vi "Generate Data_2.vi"(11 "Input":i32) -> (3 "Array out":dbl[][](array[numeric]))   [LabVIEW 2010]
panel:
  out "Waveform Graph":dbl[](graph)
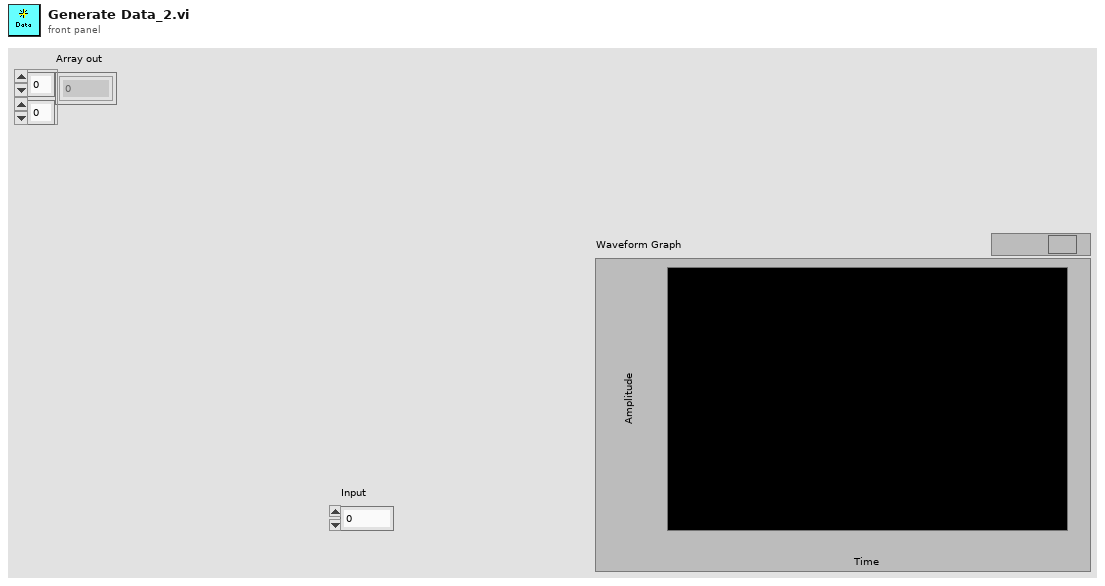
[diagram p1: front panel]
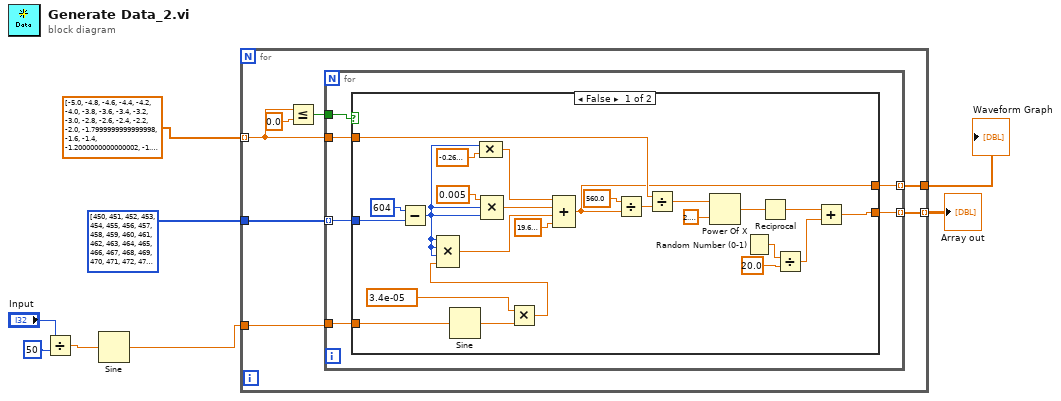
[diagram p0: block diagram]
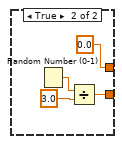
[diagram p2: hidden frame]
diagram:
  n1 = Divide(x="Input", y=50) -> (x/y=w2:dbl)
  n2 = Sine(x=w2) -> (sin(x)=w1:dbl)
  n3 = for {
    tunnel: dbl[] [-5.0, -4.8, -4.6, -4.4, -4.2, -4.0, -3.8, -3.6, -3.4, -3.2, -3.0, -2.8, -2.6, -2.4, -2.2, -2.0, -1.7999999999999998, -1.6, -1.4, -1.2000000000000002, -1.0, -0.7999999999999998, -0.5999999999999996, -0.40000000000000036, -0.20000000000000018, 0.0, 0.20000000000000018, 0.40000000000000036, 0.5999999999999996, 0.7999999999999998, 1.0, 1.2000000000000002, 1.4000000000000004, 1.5999999999999996, 1.7999999999999998, 2.0, 2.2, 2.4000000000000004, 2.5999999999999996, 2.8, 3.0, 3.1999999999999993, 3.4000000000000004, 3.5999999999999996, 3.8000000000000007, 4.0, 4.199999999999999, 4.4, 4.6, 4.800000000000001, 5.0, 5.199999999999999, 5.4, 5.6, 5.800000000000001, 6.0, 6.199999999999999, 6.4, 6.6, 6.800000000000001, 7.0, 7.199999999999999, 7.4, 7.6, 7.800000000000001, 8.0, 8.2, 8.4, 8.6, 8.8, 9.0, 9.2, 9.4, 9.6, 9.8, 10.0, 10.2, 10.4, 10.6, 10.8, 11.0, 11.2, 11.399999999999999, 11.600000000000001, 11.8, 12.0, 12.2, 12.399999999999999, 12.600000000000001, 12.8, 13.0, 13.2, 13.399999999999999, 13.600000000000001, 13.8, 14.0, 14.2, 14.399999999999999, 14.600000000000001, 14.8, 15.0, 15.2, 15.399999999999999, 15.600000000000001, 15.8, 16.0, 16.2, 16.4, 16.6, 16.8, 17.0, 17.2, 17.4, 17.6, 17.8, 18.0, 18.2, 18.4, 18.6, 18.8, 19.0, 19.2, 19.4, 19.6, 19.8, 20.0, 20.2, 20.4, 20.6, 20.8, 21.0, 21.2, 21.4, 21.6, 21.8, 22.0, 22.2, 22.4, 22.6, 22.8, 23.0, 23.2, 23.4, 23.6, 23.8, 24.0, 24.2, 24.4, 24.6, 24.8] ("Array") -> [w12] mode=indexing
    tunnel: i32[] [450, 451, 452, 453, 454, 455, 456, 457, 458, 459, 460, 461, 462, 463, 464, 465, 466, 467, 468, 469, 470, 471, 472, 473, 474, 475, 476, 477, 478, 479, 480, 481, 482, 483, 484, 485, 486, 487, 488, 489, 490, 491, 492, 493, 494, 495, 496, 497, 498, 499, 500, 501, 502, 503, 504, 505, 506, 507, 508, 509, 510, 511, 512, 513, 514, 515, 516, 517, 518, 519, 520, 521, 522, 523, 524, 525, 526, 527, 528, 529, 530, 531, 532, 533, 534, 535, 536, 537, 538, 539, 540, 541, 542, 543, 544, 545, 546, 547, 548, 549, 550, 551, 552, 553, 554, 555, 556, 557, 558, 559, 560, 561, 562, 563, 564, 565, 566, 567, 568, 569, 570, 571, 572, 573, 574, 575, 576, 577, 578, 579, 580, 581, 582, 583, 584, 585, 586, 587, 588, 589, 590, 591, 592, 593, 594, 595, 596, 597, 598, 599, 600, 601, 602, 603, 604, 605, 606, 607, 608, 609, 610, 611, 612, 613, 614, 615, 616, 617, 618, 619, 620, 621, 622, 623, 624, 625, 626, 627, 628, 629, 630, 631, 632, 633, 634, 635, 636, 637, 638, 639, 640, 641, 642, 643, 644, 645, 646, 647, 648, 649, 650, 651, 652, 653, 654, 655, 656, 657, 658, 659, 660, 661, 662, 663, 664, 665, 666, 667, 668, 669, 670, 671, 672, 673, 674, 675, 676, 677, 678, 679, 680, 681, 682, 683, 684, 685, 686, 687, 688, 689, 690, 691, 692, 693, 694, 695, 696, 697, 698, 699, 700, 701, 702, 703, 704, 705, 706, 707, 708, 709, 710, 711, 712, 713, 714, 715, 716, 717, 718, 719, 720, 721, 722, 723, 724, 725, 726, 727, 728, 729, 730, 731, 732, 733, 734, 735, 736, 737, 738, 739, 740, 741, 742, 743, 744, 745, 746, 747, 748, 749, 750, 751, 752, 753, 754, 755, 756, 757, 758, 759, 760, 761, 762, 763, 764, 765, 766, 767, 768, 769, 770, 771, 772, 773, 774, 775, 776, 777, 778, 779, 780, 781, 782, 783, 784, 785, 786, 787, 788, 789, 790, 791, 792, 793, 794, 795, 796, 797, 798, 799, 800] ("Array 2") -> [w14]
    tunnel: [w11] -> w8 mode=indexing
    tunnel: [w10] -> w7
    tunnel: w1 -> [w9]
    n4 = Less Or Equal?(x=w12, y=0.0) -> (x <= y?=w13:bool)
    n5 = for {
      tunnel: w14 -> [w18] mode=indexing
      tunnel: w13 -> [w21]
      tunnel: w12 -> [w20]
      tunnel: [w19] -> w11 mode=indexing
      tunnel: [w17] -> w10 mode=indexing
      tunnel: w9 -> [w16]
      n6 = case shown="False" w21 {
        tunnel: w20 -> [w45 _]
        tunnel: [w30 w49] -> w19
        tunnel: w18 -> [w33 _]
        tunnel: [w34 0.0] -> w17
        tunnel: w16 -> [w25 _]
        frame False {
          n7 = Subtract(x=604 ("x 2"), y=w33) -> (x-y=w32:i32)
          n8 = Sine(x=w25) -> (sin(x)=w24:dbl)
          n9 = Compound Arithmetic op=MULTIPLY(w32, -0.26000000000000006 ("c")) -> (w40:dbl)
          n10 = Compound Arithmetic op=MULTIPLY(0.005 ("b"), w32, w32) -> (w39:dbl)
          n11 = Multiply(x=3.4e-05 ("a"), y=w24) -> (x*y=w22:dbl)
          n12 = Compound Arithmetic op=MULTIPLY(w32, w32, w32, w22) -> (w38:dbl)
          n13 = Compound Arithmetic op=ADD(w40, w39, w38, 19.60000000000001 ("d")) -> (w34:dbl)
          n14 = Divide(x=560.0, y=w34) -> (x/y=w36:dbl)
          n15 = Divide(x=w45, y=w36) -> (x/y=w43:dbl)
          n16 = Power Of X(1:2.718281828459045, 2:w43) -> (0:w44:dbl)
          n17 = Random Number (0-1)() -> (number: 0 to 1=w28:dbl)
          n18 = Reciprocal(x=w44) -> (1/x=w29:dbl)
          n19 = Divide(x=w28, y=20.0) -> (x/y=w27:dbl)
          n20 = Add(x=w29, y=w27) -> (x+y=w30:dbl)
        }
        frame True {
          n21 = Random Number (0-1)() -> (number: 0 to 1=w50:dbl)
          n22 = Divide(x=w50, y=3.0) -> (x/y=w49:dbl)
        }
      }
    }
  }
  "Array out" <- w8
  "Waveform Graph" <- w7
